vi "db_begin.vi"(0 "UDL FILEPATH":path, 2 "TABLE NAME IN":string, 3 "LIST OF FIELDS?":bool, 5 "ERROR IN":errorcluster) -> (14 "REFERENCE OUT":T1, 16 "TABLE NAME OUT":string, 17 "NUMBER OF FIELDS":i32, 18 "FIELDS":string[](array[string]), 19 "Error Out":errorcluster)   [LabVIEW 2018, in "db_lib R3.lvlib"]
uses:
  db_lib R3.lvlib
  <vilib>/addons/database/Connection.llb/Conn ObjectReference.ctl
  <vilib>/addons/database/Connection.llb/DB Tools Open Connec (Path).vi
  <vilib>/addons/database/NI_Database_API.lvlib
panel:
  out "SUCCESS?":bool
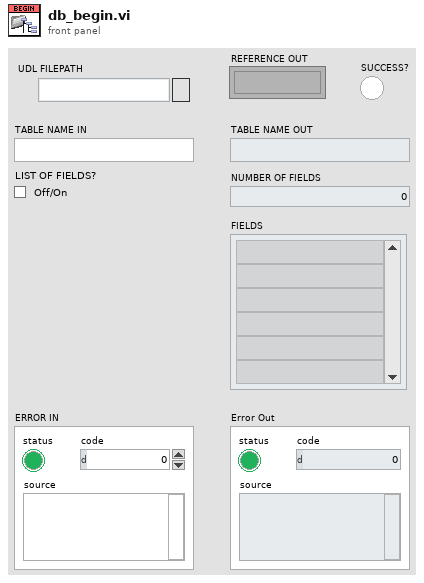
[diagram p1: front panel]
types:
  T1 = typedef "NI_Database_API.lvlib/Conn ObjectReference.ctl" = refnum<k1>
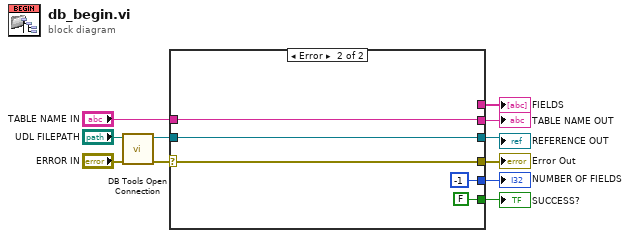
[diagram p0: block diagram]
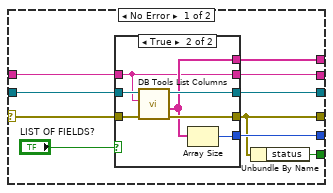
[diagram p2: hidden frame]
diagram:
  n1 = call-poly <vilib>:"DB Tools Open Connection.vi"("error in (no error)"="ERROR IN", "connection information"="UDL FILEPATH") -> ("error out"=w11:errorcluster, "connection reference"=w10:T1)  [unwired: 6 in]
  n2 = case shown="Error" w11 {
    selector: w11 -> [w20 w35]
    tunnel: w10 -> [w21 w36]
    tunnel: [w13 w35] -> w6
    tunnel: [w19 w36] -> w3
    tunnel: [w18 _] -> w7
    tunnel: [w17 -1] -> w4
    tunnel: [w15 w34] -> w5
    tunnel: "TABLE NAME IN" -> [w14 w34]
    tunnel: [w12 FALSE ("status")] -> w1
    frame No Error {
      n3 = case shown="True" "LIST OF FIELDS?" {
        tunnel: w21 -> [w23 w31]
        tunnel: w20 -> [w24 w30]
        tunnel: [w24 w29] -> w13
        tunnel: [w23 w28] -> w19
        tunnel: [_ w27] -> w18
        tunnel: [_ w26] -> w17
        tunnel: w14 -> [w22 w25]
        tunnel: [w22 w25] -> w15
        frame False {
        }
        frame True {
          n4 = call <vilib>:"DB Tools List Columns.vi"("error in (no error)"=w30, "table"=w25, "connection reference"=w31) -> ("error out"=w29:errorcluster, "columns"=w27:string[], "connection reference out"=w28:T1)  [unwired: 1 in, 1 out]
          n5 = Array Size(array=w27) -> (size(s)=w26:i32)
        }
      }
      n6 = Unbundle By Name(w13) -> ("status"=w12:bool)
    }
    frame Error {
    }
  }
  "FIELDS" <- w7
  "Error Out" <- w6
  "TABLE NAME OUT" <- w5
  "NUMBER OF FIELDS" <- w4
  "REFERENCE OUT" <- w3
  "SUCCESS?" <- w1
